vi "test Encode and Decode (Discrete).vi"(8 "error in (no error)":errorcluster, 11 "TestCase in":refnum<class "Encoding and Decoding.lvclass">) -> (0 "error out":errorcluster, 3 "TestCase out":refnum<class "Encoding and Decoding.lvclass">)   [LabVIEW 2020, in "Encoding and Decoding.lvclass"]
uses:
  Encoding and Decoding.lvclass
  Protocol/Implementations/ARINC429/Parameter Definition.ctl
  Encoding and Decoding/Encoding.ctl
  Protocol/Implementations/ARINC429/ARINC429-32bit/32-bit Word.lvclass/32-bit Word.ctl
  4413749d-09be-4b2c-9fd8-42957a21c6ba.vi
  Shared/Encode Parameter and Update Word (32-bit).vi/1445f95d-237d-4fc6-96b9-8992d347f513.vi
  Shared/Encode Parameter and Update Word (32-bit).vi/6b8853f0-8e5d-49e3-9391-4d3f8e5314b0.vi
  Shared/Encode Parameter and Update Word (32-bit).vi/2babc4f4-546e-4d35-846d-a4a1fbac0249.vi
  4413749d-09be-4b2c-9fd8-42957a21c6ba.vi/f69091ce-4ebb-4c6c-86d4-95f2f98c0ab9.vi
  4413749d-09be-4b2c-9fd8-42957a21c6ba.vi/bd4d0fb3-691f-452d-8155-40a0d56859ad.vi
  Shared/Encode Parameter and Update Word (32-bit).vi/1445f95d-237d-4fc6-96b9-8992d347f513.vi/22abf0d2-70bd-4b51-a478-b97a2704f7df.vi
  Shared/Encode Parameter and Update Word (32-bit).vi/1445f95d-237d-4fc6-96b9-8992d347f513.vi/c253b733-33bf-43c6-b07a-ea22f5c7a6f3.vi
  Shared/Encode Parameter and Update Word (32-bit).vi/1445f95d-237d-4fc6-96b9-8992d347f513.vi/9377bb8f-44b5-4a8f-87f1-966fd5a9edcc.vi
  Shared/Encode Parameter and Update Word (32-bit).vi/6b8853f0-8e5d-49e3-9391-4d3f8e5314b0.vi/a54b505c-1216-4ef4-8378-3ceda9d188df.vi
  Shared/Encode Parameter and Update Word (32-bit).vi/6b8853f0-8e5d-49e3-9391-4d3f8e5314b0.vi/136dcdcb-2dd3-4a4d-a796-a8f7a3f8e1ac.vi
  4413749d-09be-4b2c-9fd8-42957a21c6ba.vi/f69091ce-4ebb-4c6c-86d4-95f2f98c0ab9.vi/16a2565b-3c16-407b-a626-9da2a3da432e.vi
  4413749d-09be-4b2c-9fd8-42957a21c6ba.vi/bd4d0fb3-691f-452d-8155-40a0d56859ad.vi/0a001d06-2809-4638-8d0b-e017d2157007.vi
  Encoding and Decoding/BCD Decode Integer.vi
  Shared/Encode Parameter and Update Word (32-bit).vi/1445f95d-237d-4fc6-96b9-8992d347f513.vi/22abf0d2-70bd-4b51-a478-b97a2704f7df.vi/9d450a76-0fc9-4555-8e71-4c202274969f.vi
  Shared/Encode Parameter and Update Word (32-bit).vi/1445f95d-237d-4fc6-96b9-8992d347f513.vi/c253b733-33bf-43c6-b07a-ea22f5c7a6f3.vi/9d450a76-0fc9-4555-8e71-4c202274969f.vi
  Shared/Encode Parameter and Update Word (32-bit).vi/6b8853f0-8e5d-49e3-9391-4d3f8e5314b0.vi/a54b505c-1216-4ef4-8378-3ceda9d188df.vi/a7fcce85-1f75-4572-aeaa-ddfd463a7c5f.vi
  Encoding and Decoding/BCD Decode Integer.vi/9a65bfc0-0d77-4ef3-ab58-63df1e1caa90.vi
  Protocol/Implementations/ARINC429/ARINC429-32bit/32-bit Word.lvclass
  <vilib>/addons/_JKI Toolkits/VI Tester/TestCase.llb/TestCase.lvclass
  Encoding and Decoding/Encoding and Decoding.lvlib
  Protocol/Implementations/ARINC429/ARINC 429.lvclass
  C:/Program Files (x86)/National Instruments/LabVIEW 2020/vi.lib/addons/_JKI Toolkits/VI Tester/TestCase.llb/TestCase.lvclass
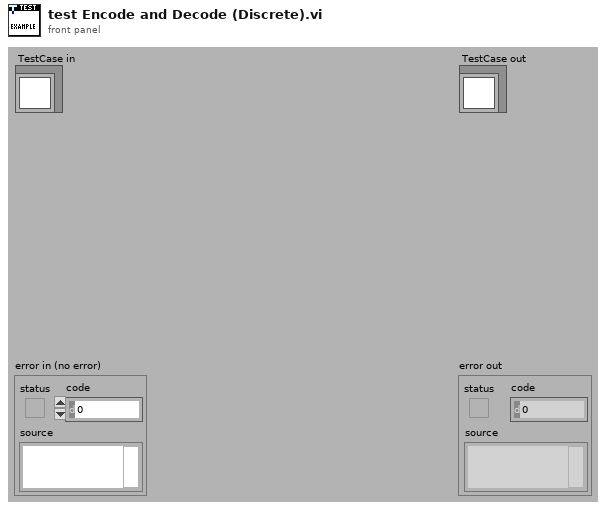
[diagram p1: front panel]
types:
  T1 = typedef "ARINC 429.lvclass/Parameter Definition.ctl" = cluster{"start index":i32, "size":i32, "encoding":T2, "signed":bool, "scale multiplier":dbl, "scale offset":dbl}
  T2 = typedef "Encoding and Decoding.lvlib/Encoding.ctl" = enum16{"BNR", "BCD", "Discrete"}
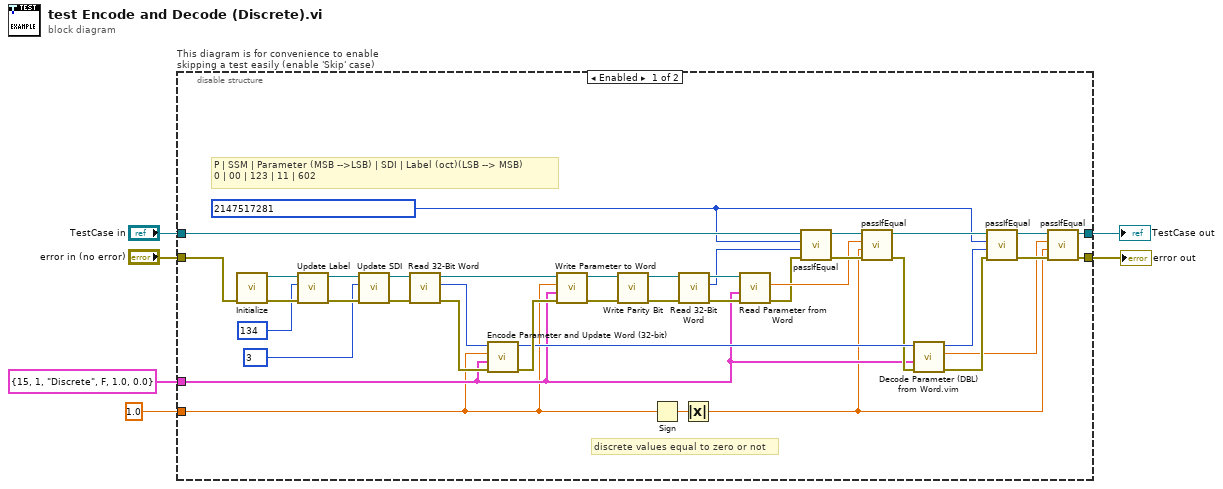
[diagram p0: block diagram]
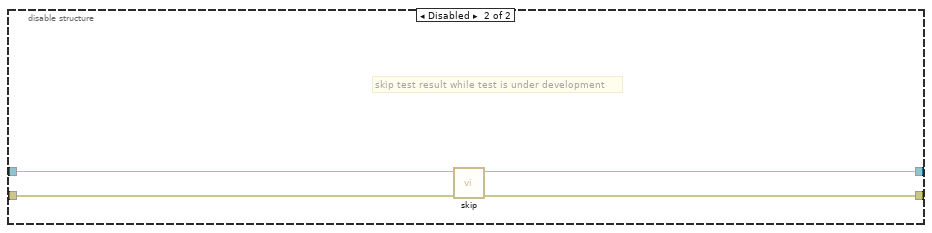
[diagram p2: hidden frame]
diagram:
  n1 = disable-structure "This diagram is for convenience to enable skipping a test easily (enable 'Skip' case)" shown="Enabled" {
    disable-tunnel: "TestCase in" -> [w29 w50]
    disable-tunnel: [w18 w48] -> w3
    disable-tunnel: [w17 w49] -> w5
    disable-tunnel: "error in (no error)" -> [w28 w47]
    disable-tunnel: T1 {"start index"=15, "size"=1, "encoding"=enum."Discrete", "signed"=FALSE, "scale multiplier"=1.0, "scale offset"=0.0} ("parameter definition") -> [w10 _]
    disable-tunnel: 1.0 ("parameter value") -> [w8 _]
    frame Enabled {
      w11 = u32 2147517281 ("SDI value 2")
      # "discrete values equal to zero or not"
      # "P | SSM | Parameter (MSB -->LSB) | SDI | Label (oct)(LSB --> MSB)\n0 | 00 | 123 | 11 | 602"
      n2 = call "Initialize.vi"("error in"=w28) -> ("error out"=w40:errorcluster, "ARINC 429 (32-bit word)"=w35:refnum<class "32-bit Word.lvclass">)  [unwired: 9 in]
      n3 = call-dynamic "Update Label.vi"("error in"=w40, "label value"=u8 134 ("label value 2"), "32-bit word in"=w35) -> ("error out"=w41:errorcluster, "32-bit word out"=w38:refnum<class "32-bit Word.lvclass">)  [unwired: 7 in]
      n4 = call-dynamic "Update SDI.vi"("error in"=w41, "SDI value"=u8 3 ("SDI value 2"), "32-bit Word in"=w38) -> ("error out"=w26:errorcluster, "32-bit Word out"=w27:refnum<class "32-bit Word.lvclass">)  [unwired: 7 in]
      n5 = call "Read 32-Bit Word.vi"("error in (no error)"=w26, "32-bit Word in"=w27) -> ("error out"=w23:errorcluster, "32-bit word"=w24:u32, "32-bit Word out"=w25:refnum<class "32-bit Word.lvclass">)  [unwired: 7 in]
      n6 = call "Encode Parameter and Update Word (32-bit).vi"("error in"=w23, "parameter definition"=w10, "parameter value"=w8, "word in"=w24) -> ("error out"=w22:errorcluster, "word out"=w21:u32)  [unwired: 6 in]
      n7 = call-dynamic "Write Parameter to Word.vi"("error in"=w22, "parameter definition"=w10, "data"=w8, "32-bit Word in"=w25) -> ("error out"=w43:errorcluster, "32-bit Word out"=w44:refnum<class "32-bit Word.lvclass">)  [unwired: 6 in]
      n8 = call-dynamic "Write Parity Bit.vi"("error in"=w43, "32-bit word in"=w44) -> ("error out"=w42:errorcluster, "32-bit word out"=w39:refnum<class "32-bit Word.lvclass">)  [unwired: 8 in]
      n9 = Sign(1:w8) -> (0:w9:dbl)
      n10 = call "Read 32-Bit Word.vi"("error in (no error)"=w42, "32-bit Word in"=w39) -> ("error out"=w46:errorcluster, "32-bit word"=w31:u32, "32-bit Word out"=w45:refnum<class "32-bit Word.lvclass">)  [unwired: 7 in]
      n11 = Absolute Value(x=w9) -> (abs(x)=w7:dbl)
      n12 = call-dynamic "Read Parameter from Word.vi"("error in"=w46, "parameter definition"=w10, "32-bit Word in"=w45) -> ("error out"=w30:errorcluster, "parameter value"=w32:dbl)  [unwired: 6 in, 1 out]
      n13 = call-dynamic "passIfEqual.vi"("error in (no error)"=w30, "y"=w31, "x"=w11, "TestCase in"=w29) -> ("error out"=w33:errorcluster, "TestCase out"=w34:refnum<class "Encoding and Decoding.lvclass">)  [unwired: 6 in]
      n14 = call-dynamic "passIfEqual.vi"("error in (no error)"=w33, "y"=w7, "x"=w32, "TestCase in"=w34) -> ("error out"=w15:errorcluster, "TestCase out"=w16:refnum<class "Encoding and Decoding.lvclass">)  [unwired: 6 in]
      n15 = call "Decode Parameter (DBL) from Word.vim"("error in"=w15, "parameter definition"=w10, "32-bit word in"=w21) -> ("error out"=w14:errorcluster, "parameter value"=w13:dbl, "32-bit word out"=w12:u32)  [unwired: 6 in]
      n16 = call-dynamic "passIfEqual.vi"("error in (no error)"=w14, "y"=w12, "x"=w11, "TestCase in"=w16) -> ("error out"=w20:errorcluster, "TestCase out"=w19:refnum<class "Encoding and Decoding.lvclass">)  [unwired: 6 in]
      n17 = call-dynamic "passIfEqual.vi"("error in (no error)"=w20, "y"=w7, "x"=w13, "TestCase in"=w19) -> ("error out"=w17:errorcluster, "TestCase out"=w18:refnum<class "Encoding and Decoding.lvclass">)  [unwired: 6 in]
    }
    frame Disabled {
      # "skip test result while test is under development"
      n18 = call <vilib>:"skip.vi"("error in (no error)"=w47, "TestCase in"=w50) -> ("error out"=w49:errorcluster, "TestCase out"=w48:refnum<class "Encoding and Decoding.lvclass">)  [unwired: 8 in]
    }
  }
  "error out" <- w5
  "TestCase out" <- w3
